vi "CALC_Fwd_adjust_TTL_pulse_length_according_to_stim_type.vi"(7 "TTL pulse length, ms in":dbl, 8 "TTL port":enum16{"TTL"}(ring), 9 "Response type":T1, 10 "Calibration parameters":T2 {"True frame time, s" format="%.10g"; "Disp. calibration info"."Speed, µl per ms" format="%.3g"; "True FPS" format="%.10g"; "Timing calibration sw/hw" format="%.10g"}, 11 "TTL pulse length ref in":refnum<vi>) -> (3 "TTL pulse length, ms out":dbl)   [LabVIEW 2018, in "Tracker.lvlib"]
uses:
  Tracker.lvlib
  Controls/CTL_Calibration_parameters.ctl
  Controls/CTL_Dispenser_calibration_info.ctl
  Controls/CTL_Condition_response_type.ctl
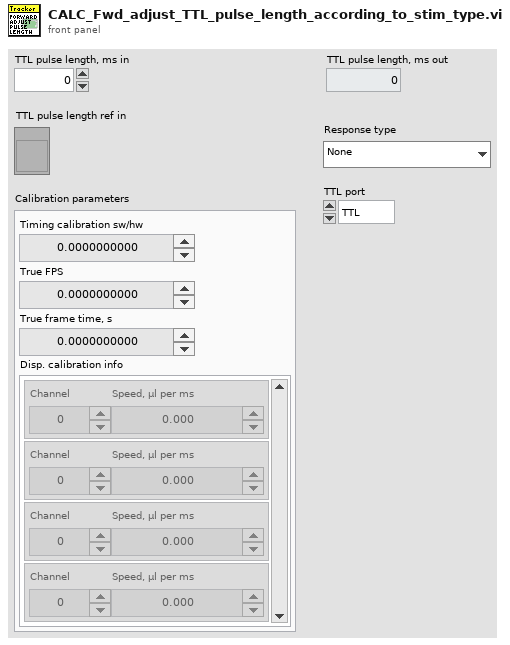
[diagram p1: front panel]
types:
  T1 = typedef "Tracker.lvlib/CTL_Condition_response_type.ctl" = enum16{"None", "Air puff", "Liquid reward"}
  T2 = typedef "Tracker.lvlib/CTL_Calibration_parameters.ctl" = cluster{"Timing calibration sw/hw":dbl, "True FPS":dbl, "True frame time, s":dbl, "Disp. calibration info":T3}
  T3 = typedef "Tracker.lvlib/CTL_Dispenser_calibration_info.ctl" = cluster{"Channel":u8, "Speed, µl per ms":dbl}[]
  T4 = enum8{"Enabled", "Disabled", "Disabled and Grayed Out"}
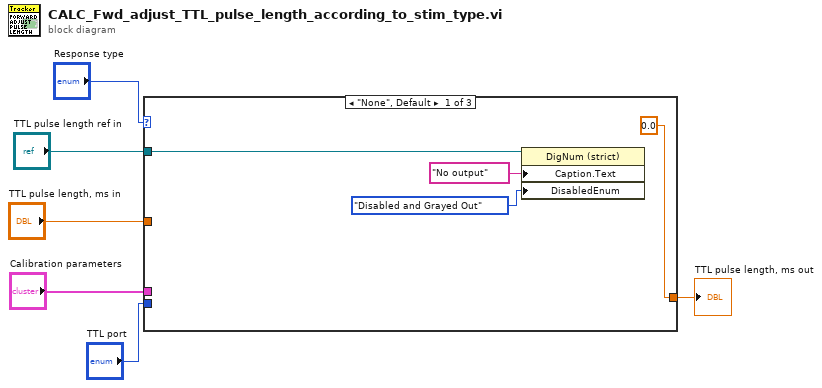
[diagram p0: block diagram]
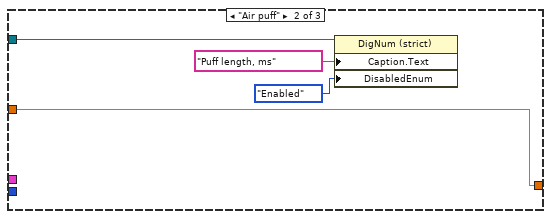
[diagram p2: hidden frame]
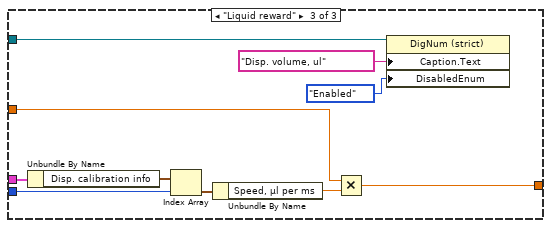
[diagram p3: hidden frame]
diagram:
  n1 = case shown="\"None\", Default" "Response type" {
    tunnel: [0.0 ("TTL pulse length, ms") w14 w18] -> w3
    tunnel: "TTL pulse length, ms in" -> [_ w14 w19]
    tunnel: "Calibration parameters" -> [_ _ w24]
    tunnel: "TTL port" -> [_ _ w22]
    tunnel: "TTL pulse length ref in" -> [w7 w11 w15]
    frame "None", Default {
      n2 = property on="Property Node" class="DigNum (strict)"(reference=w7, "Caption.Text"="No output", "DisabledEnum"=T4."Disabled and Grayed Out" ("Disabled")) -> ()  [unwired: 1 in, 2 out]
    }
    frame "Air puff" {
      n3 = property on="Property Node" class="DigNum (strict)"(reference=w11, "Caption.Text"="Puff length, ms", "DisabledEnum"=T4."Enabled" ("Disabled")) -> ()  [unwired: 1 in, 2 out]
    }
    frame "Liquid reward" {
      n4 = Unbundle By Name(w24) -> ("Disp. calibration info"=w23:T3)
      n5 = Index Array(array=w23, index=w22) -> (element=w21:cluster{"Channel":u8, "Speed, µl per ms":dbl})
      n6 = Unbundle By Name(w21) -> ("Speed, µl per ms"=w20:dbl)
      n7 = Multiply(x=w19, y=w20) -> (x*y=w18:dbl)
      n8 = property on="Property Node" class="DigNum (strict)"(reference=w15, "Caption.Text"="Disp. volume, ul", "DisabledEnum"=T4."Enabled" ("Disabled")) -> ()  [unwired: 1 in, 2 out]
    }
  }
  "TTL pulse length, ms out" <- w3
